vi "Perform Action.vi"(8 "error in":errorcluster, 10 "Input":variant, 11 "HSU MCU V2 in":refnum<class "HSU MCU V2 CFG.lvclass">) -> (0 "error out":errorcluster, 2 "Output":variant, 3 "HSU MCU V2 out":refnum<class "HSU MCU V2 CFG.lvclass">)   [LabVIEW 2023, in "HSU MCU V2 CFG.lvclass"]
uses:
  HSU MCU V2 CFG.lvclass
  Attribute Selector.ctl
  MCU Selector.ctl
  HSU MCU V2 CFG.lvclass/HSU MCU V2 CFG.ctl
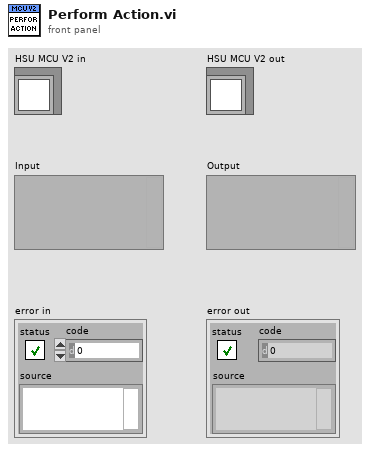
[diagram p1: front panel]
types:
  T1 = typedef "MCU Selector.ctl" = enum16{"Default", "MCU1", "MCU2", "MCU3", "MCU4", "MCU5", "MCU6", "MCU7", "MCU8"}
  T2 = typedef "Attribute Selector.ctl" = enum16{"MCU_FAULT", "MCU_STATE", "MCU_Temp_Winding", "MCU_Temp_PowerStage", "MCU_Speed", "MCU_I_REF", "MCU_ENABLE", "MCU_U_DC", "Power", "Torque"}
  T3 = cluster{"Action":enum16{"Read", "Write"}, "MCU":string, "Attribute":string, "Value":variant}
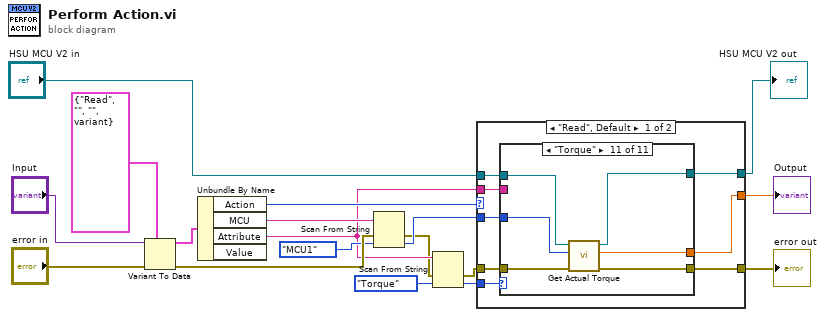
[diagram p0: block diagram]
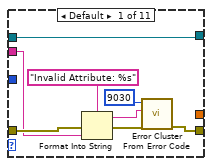
[diagram p2: hidden frame]
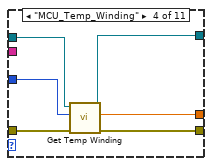
[diagram p5: hidden frame]
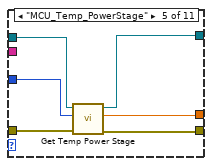
[diagram p6: hidden frame]
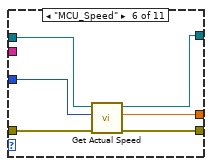
[diagram p7: hidden frame]
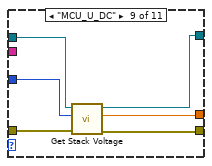
[diagram p10: hidden frame]
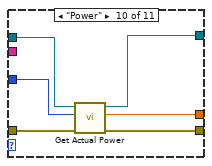
[diagram p11: hidden frame]
diagram:
  n1 = Variant To Data(error in="error in", type=T3 {"Action"=enum."Read", "MCU"="", "Attribute"="", "Value"=variant}, Variant="Input") -> (data=w1:T3, error out=w14:errorcluster)
  n2 = Unbundle By Name(w1) -> ("Action"=w17:enum16{"Read", "Write"}, "MCU"=w7:string, "Attribute"=w4:string)  [unwired: 1 out]
  n3 = Scan From String(input string=w7, error in=w14, default 1=MCU_Selector."MCU1" ("MCU Selector")) -> (error out=w3:errorcluster, output 1=w5:T1)  [unwired: 2 in, 2 out]
  n4 = Scan From String(input string=w4, error in=w3, default 1=Attribute_Selector."Torque") -> (error out=w9:errorcluster, output 1=w8:T2)  [unwired: 2 in, 2 out]
  n5 = case shown="\"Read\", Default" w17 {
    tunnel: "HSU MCU V2 in" -> [w26 w79]
    tunnel: [w25 w80] -> w16
    tunnel: [w24 _] -> w13
    tunnel: [w23 w79] -> w11
    tunnel: w9 -> [w22 w80]
    tunnel: w8 -> [w21 _]
    tunnel: w5 -> [w20 _]
    tunnel: w4 -> [w19 _]
    frame "Read", Default {
      n6 = case shown="\"Torque\"" w21 {
        tunnel: w22 -> [w31 w35 w38 w44 w50 w56 w57 w59 w66 w72 w78]
        tunnel: w26 -> [w29 w36 w37 w42 w48 w52 w58 w60 w64 w69 w76]
        tunnel: [w34 w35 w38 w39 w45 w55 w57 w59 w63 w71 w77] -> w25
        tunnel: [_ _ _ w40 w46 w53 _ _ w62 w70 w74] -> w24
        tunnel: [w29 w36 w37 w41 w47 w51 w58 w60 w61 w68 w75] -> w23
        tunnel: w20 -> [_ _ _ w43 w49 w54 _ _ w65 w67 w73]
        tunnel: w19 -> [w28 _ _ _ _ _ _ _ _ _ _]
        frame Default {
          n7 = Format Into String(format string="Invalid Attribute: %s" ("error message (\"\")"), error in=w31, w28) -> (resulting string=w33:string, error out=w30:errorcluster)  [unwired: 1 in]
          n8 = call <vilib>:"Error Cluster From Error Code.vi"("error in (no error)"=w30, "error message (\"\")"=w33, "error code (0)"=9030) -> ("error out"=w34:errorcluster)  [unwired: 6 in]
        }
        frame "MCU_FAULT" {
        }
        frame "MCU_STATE" {
        }
        frame "MCU_Temp_Winding" {
          n9 = call "Get Temp Winding.vi"("error in"=w44, "MCU Selector"=w43, "HSU MCU V2 Monitor CFG in"=w42) -> ("error out"=w39:errorcluster, "Temperature"=w40:dbl, "HSU MCU V2 Monitor CFG out"=w41:refnum<class "HSU MCU V2 CFG.lvclass">)  [unwired: 6 in]
        }
        frame "MCU_Temp_PowerStage" {
          n10 = call "Get Temp Power Stage.vi"("error in"=w50, "MCU Selector"=w49, "HSU MCU V2 Monitor CFG in"=w48) -> ("error out"=w45:errorcluster, "Temperature"=w46:dbl, "HSU MCU V2 Monitor CFG out"=w47:refnum<class "HSU MCU V2 CFG.lvclass">)  [unwired: 6 in]
        }
        frame "MCU_Speed" {
          n11 = call "Get Actual Speed.vi"("error in"=w56, "MCU Selector"=w54, "HSU MCU V2 Monitor CFG in"=w52) -> ("error out"=w55:errorcluster, "Speed"=w53:dbl, "HSU MCU V2 Monitor CFG out"=w51:refnum<class "HSU MCU V2 CFG.lvclass">)  [unwired: 6 in]
        }
        frame "MCU_I_REF" {
        }
        frame "MCU_ENABLE" {
        }
        frame "MCU_U_DC" {
          n12 = call "Get Stack Voltage.vi"("error in"=w66, "MCU Selector"=w65, "HSU MCU V2 Monitor CFG in"=w64) -> ("error out"=w63:errorcluster, "Voltage DC"=w62:dbl, "HSU MCU V2 Monitor CFG out"=w61:refnum<class "HSU MCU V2 CFG.lvclass">)  [unwired: 6 in]
        }
        frame "Power" {
          n13 = call "Get Actual Power.vi"("error in"=w72, "MCU Selector"=w67, "HSU MCU V2 CFG in"=w69) -> ("error out"=w71:errorcluster, "Power"=w70:dbl, "HSU MCU V2 CFG out"=w68:refnum<class "HSU MCU V2 CFG.lvclass">)  [unwired: 5 in, 1 out]
        }
        frame "Torque" {
          n14 = call "Get Actual Torque.vi"("error in"=w78, "MCU Selector"=w73, "HSU MCU V2 Monitor CFG in"=w76) -> ("error out"=w77:errorcluster, "Torque"=w74:dbl, "HSU MCU V2 Monitor CFG out"=w75:refnum<class "HSU MCU V2 CFG.lvclass">)  [unwired: 6 in]
        }
      }
    }
    frame "Write" {
    }
  }
  "error out" <- w16
  "HSU MCU V2 out" <- w11
  "Output" <- w13
